vi "SICK Only Init.vi"(7 "SICK Init Timeout":i32=2000, 8 "error in":errorcluster, 10 "SICK Commands":string[][](array[string]), 11 "SICK Only ref in":T1) -> (0 "error out":errorcluster, 2 "Init Success":bool, 3 "SICK Only ref out":T1)   [LabVIEW 2009]
uses:
  SICK Only FPGA Ref.ctl
  <vilib>/rvi/interface/nirviReadWriteControl/nirviReadWriteControl.xnode
  FPGA Bitfiles/Q_IGVC_2010.lvproj_FPGA Target_SICK Only.vi.lvbitx
  <vilib>/Utility/error.llb/Error Cluster From Error Code.vi
  <vilib>/rvi/errors/niLvFpgaAdjustHostInterfaceError.vi
  <vilib>/rvi/interface/common/niFpgaNodeNameForErrorReporting.ctl
  <vilib>/rvi/errors/niLvFpgaWhatHappensToTopLevelVI.ctl
  <vilib>/rvi/interface/nirviMethod/nirviMethod.xnode
  <vilib>/LabVIEW Targets/FPGA/RIO/nirio_HostInterface/nirio_WaitOnIRQ.vi
  <vilib>/RVI Host/nirviSupport.llb/nirviErrorClusterFromErrorCode.vi
  NiRioSrv.dll
panel:
  out "Initialization success":bool
  out "Commands":u8[](array[numeric])=[8, 2, 0, 2, 0, 32, 36, 52, 8, 0, 0, 0, 0, 0, 0, 0, 0, 7, 6, 2, 128, 3, 0, 160, 0, 0, 0, 0, 0, 0, 0, 0] format="%x"
  out "Response":u8[](array[numeric])=[6, 2, 128, 3, 0, 160, 0] format="%x"
  out "Command":u8[](array[numeric])=[2, 0, 2, 0, 32, 36, 52, 8] format="%x"
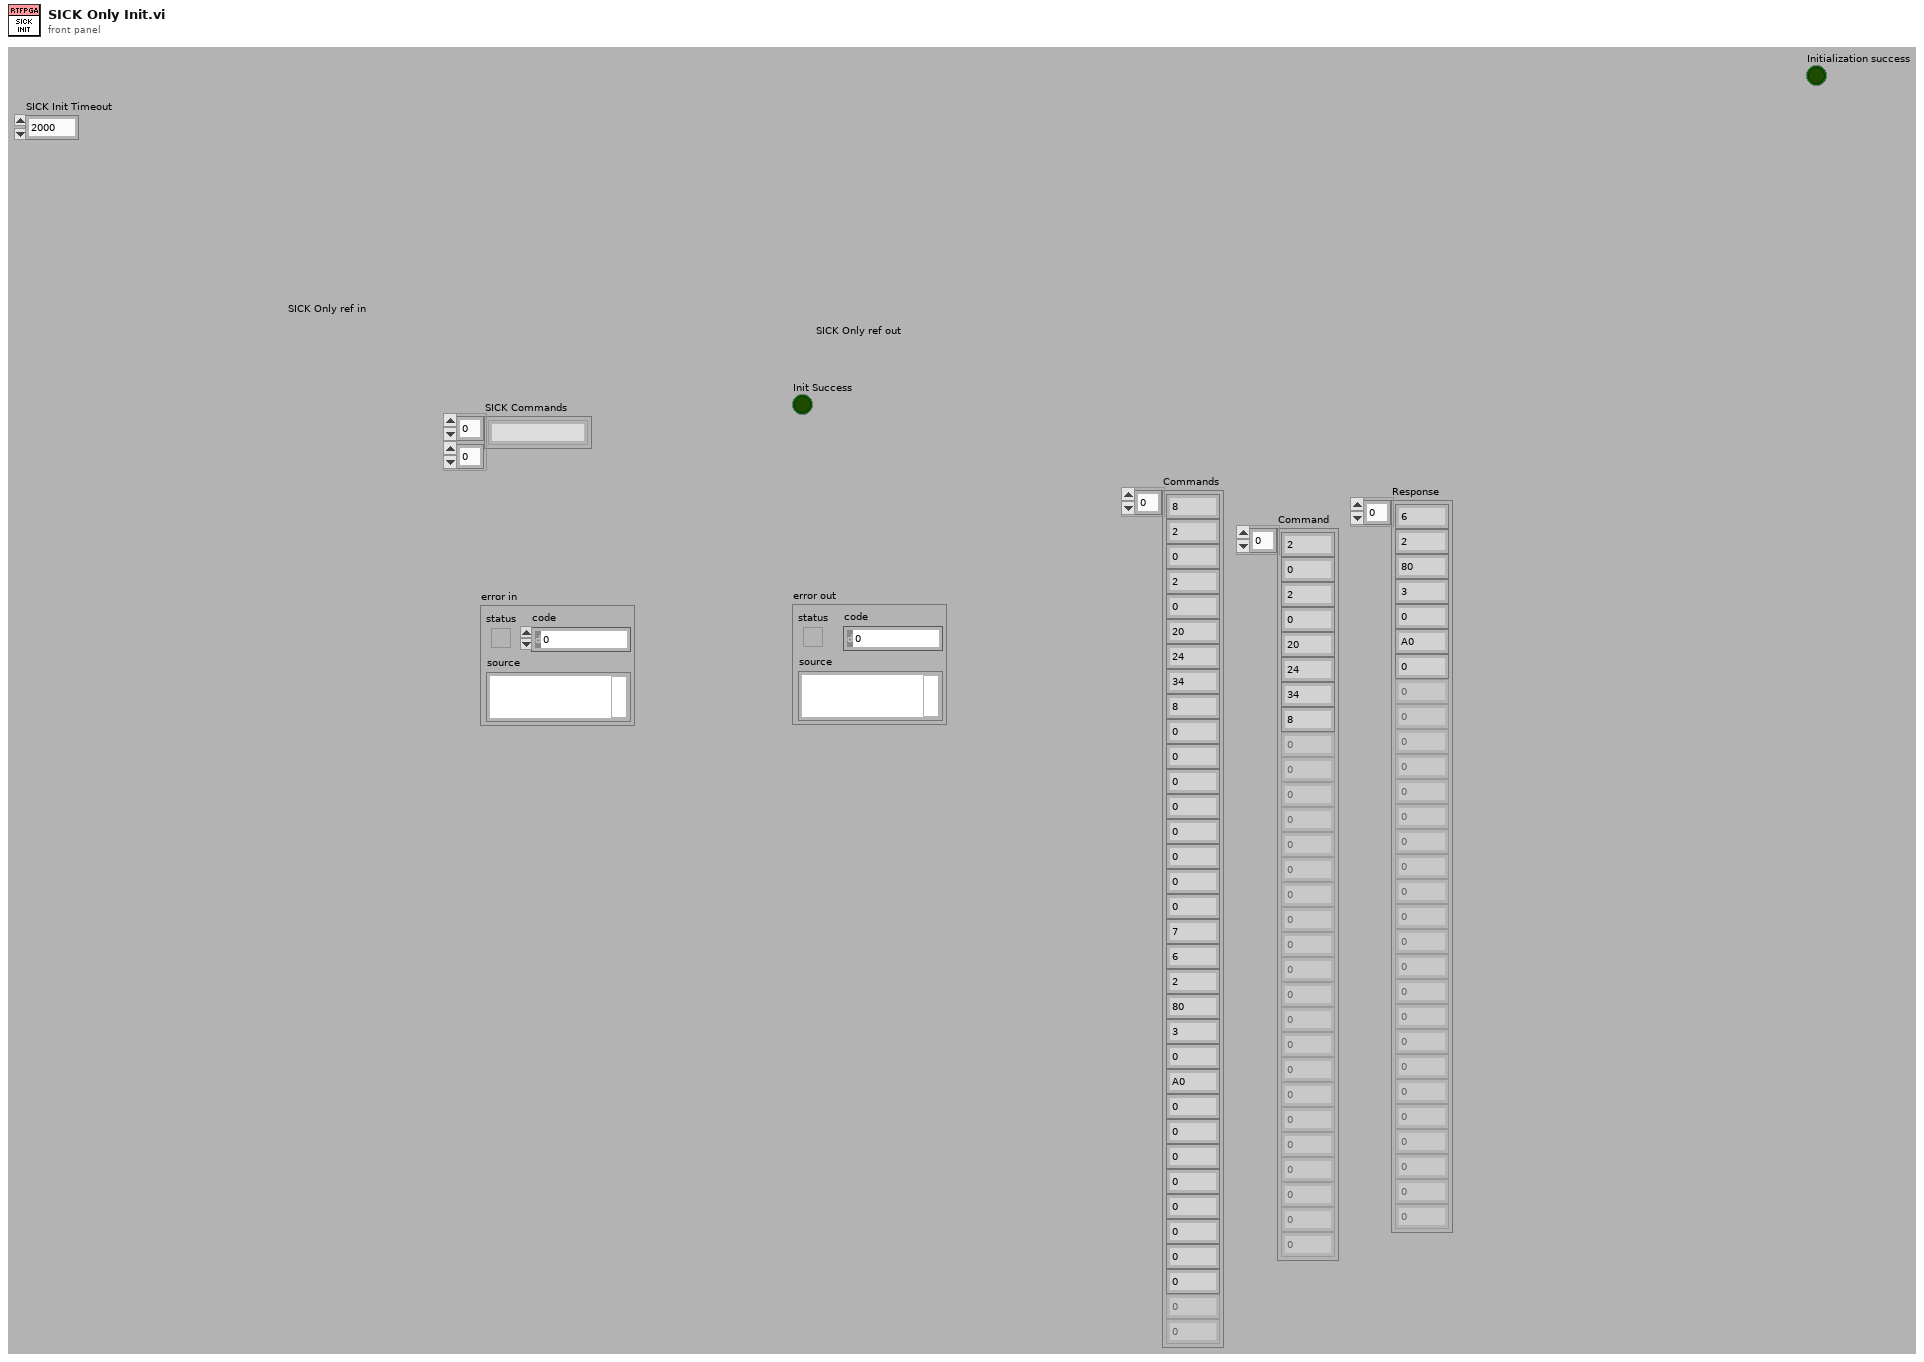
[diagram p1: front panel]
types:
  T1 = typedef "SICK Only FPGA Ref.ctl" = refnum<k20>
  T2 = typedef "niFpgaNodeNameForErrorReporting.ctl" = enum16{"Open FPGA VI Reference", "Read/Write Control", "Invoke Method: Abort", "Invoke Method: Acknowledge IRQ", "Invoke Method: Download", "Invoke Method: FIFO.Configure", "Invoke Method: FIFO.Read", "Invoke Method: FIFO.Start", "Invoke Method: FIFO.Stop", "Invoke Method: FIFO.Write", "Invoke Method: Reset", "Invoke Method: Run", "Invoke Method: Wait on IRQ", "Close FPGA VI Reference"}
  T3 = typedef "niLvFpgaWhatHappensToTopLevelVI.ctl" = enum16{"top level VI scripted behind XNode", "top level VI inlined behind XNode"}
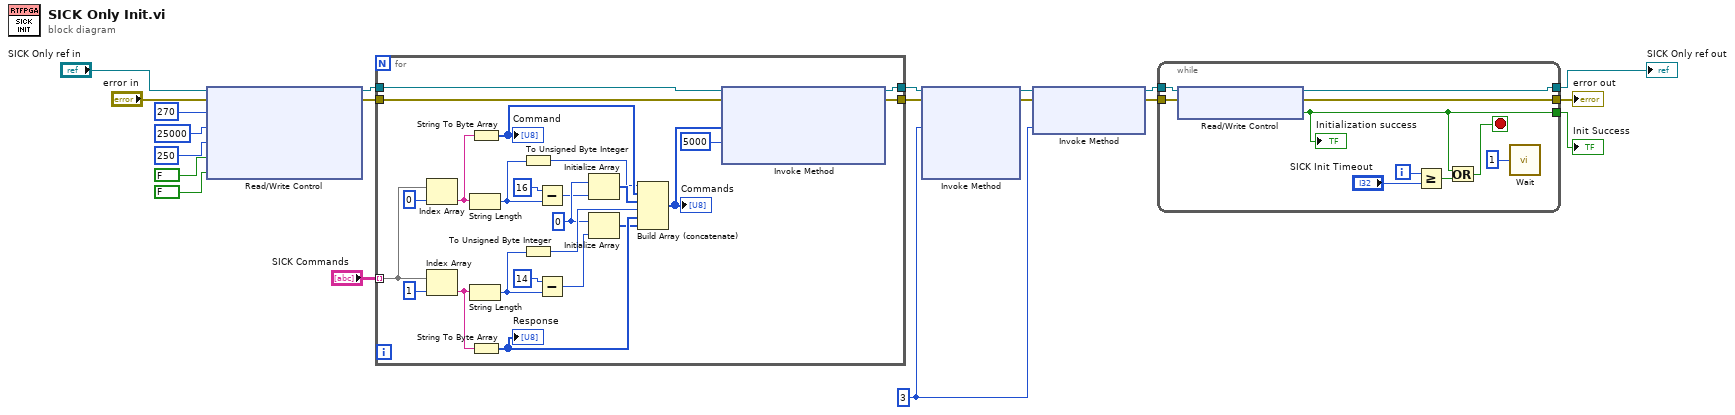
[diagram p0: block diagram]
diagram:
  w4 = 3 ("IRQ Number(s)")
  n1 = xnode "Read/Write Control"("FPGA VI Reference In"="SICK Only ref in", "error in"="error in", "Overflow Reading"=u16 270, "Bytes at Port Timeout (us)"=25000, "Read/Write Timeout (ms)"=250, "En overflow replacement"=FALSE, "EN mask overflow bytes"=FALSE) -> ("FPGA VI Reference Out"=w11:T1, "error out"=w10:errorcluster)
  n2 = for {
    tunnel: [w39] -> w3
    tunnel: [w38] -> w2
    tunnel: "SICK Commands" -> [w23] mode=indexing
    tunnel: w11 -> [w22]
    tunnel: w10 -> [w21]
    w32 = u8 0 ("index")
    n3 = Index Array(array=w23, index=0) -> (element=w42:string)
    n4 = Index Array(array=w23, index=1) -> (element=w40:string)
    n5 = String Length(string=w42) -> (length=w30:i32)
    n6 = String Length(string=w40) -> (length=w25:i32)
    n7 = String To Byte Array(string=w42) -> (unsigned byte array=w41:u8[])
    "Command" <- w41
    n8 = String To Byte Array(string=w40) -> (unsigned byte array=w36:u8[])
    "Response" <- w36
    n9 = To Unsigned Byte Integer(number=w30) -> (unsigned 8bit integer=w31:u8)
    n10 = To Unsigned Byte Integer(number=w25) -> (unsigned 8bit integer=w35:u8)
    n11 = Subtract(x=16 ("y"), y=w30) -> (x-y=w28:i32)
    n12 = Subtract(x=14 ("y"), y=w25) -> (x-y=w27:i32)
    n13 = Initialize Array(w32, w28) -> (w33:u8[])
    n14 = Initialize Array(w32, w27) -> (w34:u8[])
    n15 = Build Array (concatenate)(w31, w41, w33, w35, w36, w34) -> (w37:u8[])
    "Commands" <- w37
    n16 = xnode "Invoke Method"("FPGA VI Reference In"=w22, "error in"=w21, "Data"=w37, "Timeout (ms)"=5000) -> ("FPGA VI Reference Out"=w39:T1, "error out"=w38:errorcluster)  [unwired: 1 out]
  }
  n17 = xnode "Invoke Method"("FPGA VI Reference In"=w3, "error in"=w2, "IRQ Number(s)"=w4) -> ("FPGA VI Reference Out"=w5:T1, "error out"=w6:errorcluster)  [unwired: 3 out]
  n18 = xnode "Invoke Method"("FPGA VI Reference In"=w5, "error in"=w6, "IRQ Number(s)"=w4) -> ("FPGA VI Reference Out"=w13:T1, "error out"=w12:errorcluster)
  n19 = while {
    tunnel: w13 -> [w120]
    tunnel: [w117] -> w8
    tunnel: w12 -> [w119]
    tunnel: [w118] -> w9
    tunnel: [w111] -> w7
    i -> [w115]
    stop <- w113 stop-if-true
    n20 = xnode "Read/Write Control"("FPGA VI Reference In"=w120, "error in"=w119) -> ("FPGA VI Reference Out"=w118:T1, "error out"=w117:errorcluster, "Initialization success"=w111:bool)
    "Initialization success" <- w111
    n21 = Greater Or Equal?(x=w115, y="SICK Init Timeout") -> (x >= y?=w112:bool)
    n22 = Or(x=w111, y=w112) -> (x .or. y?=w113:bool)
    n23 = call "Wait"("Count(mSec)"=u32 1 ("milliseconds to wait")) -> ()  [unwired: 1 out]
  }
  "SICK Only ref out" <- w9
  "error out" <- w8
  "Init Success" <- w7
